vi "Library Wildcards to Regular.vi"(4 "wildcards":string) -> (1 "regular expression":string)   [LabVIEW 2012]
doc: "Converts a string holding '*' and '?' wildcards into an equivalent LabVIEW regular expression that can be passed into match pattern. Useful for filter strings in user interfaces: users are often familiar with wildcards but not with regular expressions. \n\nNote that the match will be case-dependent unless you make is case-independent by converting the regular expression and string to be matched to all lower or all upper case."
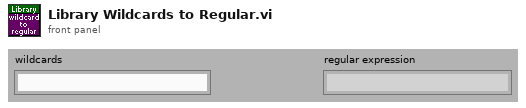
[diagram p1: front panel]
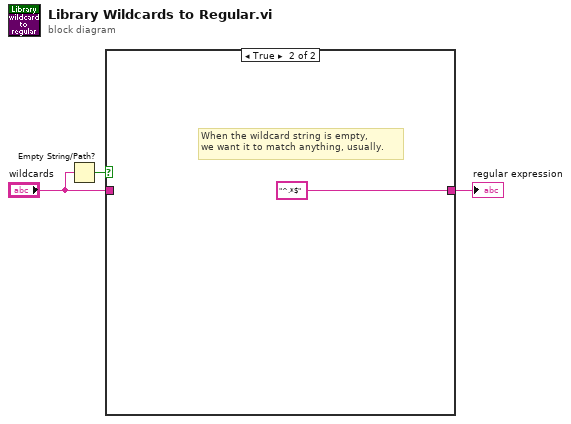
[diagram p0: block diagram]
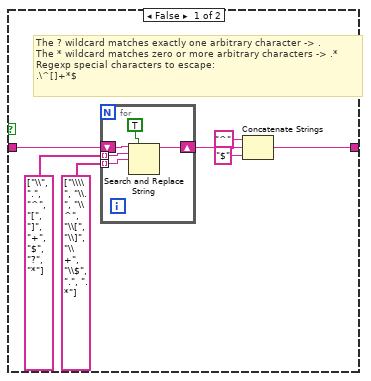
[diagram p2: hidden frame]
diagram:
  n1 = Empty String/Path?(string/path="wildcards") -> (empty?=w3:bool)
  n2 = case shown="True" w3 {
    tunnel: "wildcards" -> [w10 _]
    tunnel: [w5 "^.*$"] -> w1
    frame False {
      # "The ? wildcard matches exactly one arbitrary character -> .\nThe * wildcard matches zero or more arbitrary characters -> .*\nRegexp special characters to escape:\n.\\^[]+*$"
      n3 = for {
        shift-right: [w14] -> w7
        shift-left: w10 -> [w15]
        tunnel: string[] ["\\", ".", "^", "[", "]", "+", "$", "?", "*"] -> [w12] mode=indexing
        tunnel: string[] ["\\\\", "\\.", "\\^", "\\[", "\\]", "\\+", "\\$", ".", ".*"] -> [w11] mode=indexing
        n4 = Search and Replace String(replace all?=TRUE ("replace all? (F)"), input string=w15, search string=w12, replace string=w11) -> (result string=w14:string)  [unwired: 4 in, 3 out]
      }
      n5 = Concatenate Strings("^" ("string"), w7, "$" ("string")) -> (w5:string)
    }
    frame True {
      # "When the wildcard string is empty,\nwe want it to match anything, usually."
    }
  }
  "regular expression" <- w1
